vi "Set Protocol Data.vi"(7 "Operation":T1, 8 "error in (no error)":errorcluster, 10 "Protocols.lvlib:Protocol Parent.lvclass":refnum<class "Protocol Parent.lvclass">, 11 "Listener In.lvclass":refnum<class "Listener.lvclass"> caption="Listener") -> (0 "error out":errorcluster, 3 "Listener Out.lvclass":refnum<class "Listener.lvclass">)   [LabVIEW 2019, in "Listener.lvclass"]
uses:
  Listener.lvclass
  Protocol Parent/Protocol Parent.lvclass
  ListenerClassControls/Operation.ctl
  AK TCP/AK TCP.lvclass
  D:/GitRepository/niveristand-instrument-addon-classes/Source/Protocols/TCP/TCP.lvclass
  ListenerClassControls/AK TCP Data Structure.ctl
  ListenerClassControls/Protocol.ctl
  TCP/TCP.lvclass/TCP.ctl
  TCP/TCP.lvclass
  ListenerClassControls/TCP Data Structure.ctl
  UDP/UDP.lvclass
  ListenerClassControls/UDP Data Structure.ctl
  UDP/UDP.lvclass/UDP.ctl
  ListenerClassControls/VISA Data Structure.ctl
  AK RS-xxx/AK RS-xxx.lvclass
  ListenerClassControls/RS-xxx Data Structure.ctl
  ListenerClassControls/RS-xxx To GPIB ConvBox Data Structure.ctl
  TCP/Data Access/Read IP Address.vi
  TCP/Data Access/Read Port.vi
  UDP/Data Access/Read Target IP Address.vi
  UDP/Data Access/Read Local Port.vi
  UDP/Data Access/Read Local IP Address.vi
  UDP/Data Access/Read Target Port.vi
  Constants.vi
  <vilib>/Instr/_visa.llb/VISA Configure Serial Port (Instr).vi
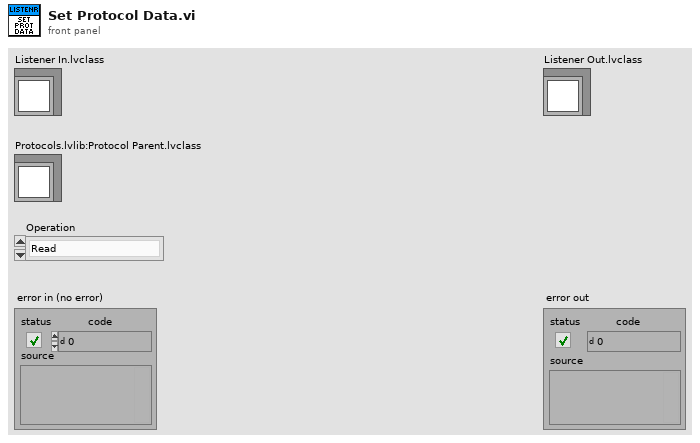
[diagram p1: front panel]
types:
  T1 = typedef "Listener.lvclass/Operation.ctl" = enum16{"Read", "Write"}
  T2 = typedef "Listener.lvclass/Protocol.ctl" = enum16{"RS-XXX", "AK RS-XXX", "VISA", "TCPIP", "AK TCPIP", "UDP", "GPIB ConvBox"}
  T3 = typedef "Listener.lvclass/AK TCP Data Structure.ctl" = cluster{"TCP|IP connection ID":refnum<k5>, "IP Address":string, "Port":u16, "Data":string, "Current Command Code":string}
  T4 = typedef "Listener.lvclass/TCP Data Structure.ctl" = cluster{"TCP|IP connection ID":refnum<k5>, "IP Address":string, "Port":u16, "Data":string}
  T5 = typedef "Listener.lvclass/UDP Data Structure.ctl" = cluster{"UDP connection ID":refnum<k16>, "Local Address":string, "Local Port":u16, "Target IP Address":string, "Target Port":u16, "Data":string}
  T6 = typedef "Listener.lvclass/VISA Data Structure.ctl" = cluster{"Protocol Ref Out":refnum<visa-resource-name>, "Listener Ref Out":refnum<visa-resource-name>, "Data Length":u32, "Data":string}
  T7 = typedef "Listener.lvclass/RS-xxx Data Structure.ctl" = cluster{"Listener Port Ref":refnum<visa-resource-name>, "Protocol Port Ref":refnum<visa-resource-name>, "Virtual COM Port Settings 1":cluster{"Port":string, "Baud Rate":u32, "Data Bits":u16, "Parity":enum16{"None", "Odd", "Even", "Mark", "Space"}, "Stop Bits":u16, "Flow Control":u16, "XON":enum16{"NUL", "SOH", "STX", "ETX", "EOT", "ENQ", "ACK", "BEL", "BS", "HT", "LF", "VT", "FF", "CR", "SO", "SI", "DLE", "DC1", "DC2", "DC3", "DC4", "NAK", "SYN", "ETB", "CAN", "EM", "SUB", "ESC", "FS", "GS", "RS", "US", "SP", "!", "\"", "#", "$", "%", "&", "'", "(", ")", "*", "+", ",", "- (-)", ".", "/", "0", "1", "2", "3", "4", "5", "6", "7", "8", "9", ":", ";", "<", "=", ">", "?", "@", "A", "B", "C", "D", "E", "F", "G", "H", "I", "J", "K", "L", "M", "N", "O", "P", "Q", "R", "S", "T", "U", "V", "W", "X", "Y", "Z", "[", "\\", "]", "^", "_", "`", "a", "b", "c", "d", "e", "f", "g", "h", "i", "j", "k", "l", "m", "n", "o", "p", "q", "r", "s", "t", "u", "v", "w", "x", "y", "z", "{", "|", "}", "~"}, "XOFF":enum16{"NUL", "SOH", "STX", "ETX", "EOT", "ENQ", "ACK", "BEL", "BS", "HT", "LF", "VT", "FF", "CR", "SO", "SI", "DLE", "DC1", "DC2", "DC3", "DC4", "NAK", "SYN", "ETB", "CAN", "EM", "SUB", "ESC", "FS", "GS", "RS", "US", "SP", "!", "\"", "#", "$", "%", "&", "'", "(", ")", "*", "+", ",", "- (-)", ".", "/", "0", "1", "2", "3", "4", "5", "6", "7", "8", "9", ":", ";", "<", "=", ">", "?", "@", "A", "B", "C", "D", "E", "F", "G", "H", "I", "J", "K", "L", "M", "N", "O", "P", "Q", "R", "S", "T", "U", "V", "W", "X", "Y", "Z", "[", "\\", "]", "^", "_", "`", "a", "b", "c", "d", "e", "f", "g", "h", "i", "j", "k", "l", "m", "n", "o", "p", "q", "r", "s", "t", "u", "v", "w", "x", "y", "z", "{", "|", "}", "~"}, "End Read on Termination Character":bool, "End Write on Termination Character":bool, "Termination Character":u8}, "Virtual COM Port Settings 2":cluster{"Port":string, "Baud Rate":u32, "Data Bits":u16, "Parity":enum16{"None", "Odd", "Even", "Mark", "Space"}, "Stop Bits":u16, "Flow Control":u16, "XON":enum16{"NUL", "SOH", "STX", "ETX", "EOT", "ENQ", "ACK", "BEL", "BS", "HT", "LF", "VT", "FF", "CR", "SO", "SI", "DLE", "DC1", "DC2", "DC3", "DC4", "NAK", "SYN", "ETB", "CAN", "EM", "SUB", "ESC", "FS", "GS", "RS", "US", "SP", "!", "\"", "#", "$", "%", "&", "'", "(", ")", "*", "+", ",", "- (-)", ".", "/", "0", "1", "2", "3", "4", "5", "6", "7", "8", "9", ":", ";", "<", "=", ">", "?", "@", "A", "B", "C", "D", "E", "F", "G", "H", "I", "J", "K", "L", "M", "N", "O", "P", "Q", "R", "S", "T", "U", "V", "W", "X", "Y", "Z", "[", "\\", "]", "^", "_", "`", "a", "b", "c", "d", "e", "f", "g", "h", "i", "j", "k", "l", "m", "n", "o", "p", "q", "r", "s", "t", "u", "v", "w", "x", "y", "z", "{", "|", "}", "~"}, "XOFF":enum16{"NUL", "SOH", "STX", "ETX", "EOT", "ENQ", "ACK", "BEL", "BS", "HT", "LF", "VT", "FF", "CR", "SO", "SI", "DLE", "DC1", "DC2", "DC3", "DC4", "NAK", "SYN", "ETB", "CAN", "EM", "SUB", "ESC", "FS", "GS", "RS", "US", "SP", "!", "\"", "#", "$", "%", "&", "'", "(", ")", "*", "+", ",", "- (-)", ".", "/", "0", "1", "2", "3", "4", "5", "6", "7", "8", "9", ":", ";", "<", "=", ">", "?", "@", "A", "B", "C", "D", "E", "F", "G", "H", "I", "J", "K", "L", "M", "N", "O", "P", "Q", "R", "S", "T", "U", "V", "W", "X", "Y", "Z", "[", "\\", "]", "^", "_", "`", "a", "b", "c", "d", "e", "f", "g", "h", "i", "j", "k", "l", "m", "n", "o", "p", "q", "r", "s", "t", "u", "v", "w", "x", "y", "z", "{", "|", "}", "~"}, "End Read on Termination Character":bool, "End Write on Termination Character":bool, "Termination Character":u8}, "Data":string, "Data Length":u32}
  T8 = typedef "Listener.lvclass/RS-xxx To GPIB ConvBox Data Structure.ctl" = cluster{"Protocol Port Ref":refnum<visa-resource-name>, "Listener Port Ref":refnum<visa-resource-name>, "Data":string, "Command Messages Read":string[], "Address":string}
  T9 = typedef "Protocols.lvlib/Protocol Parent.lvclass/Base Protocol Type.ctl" = enum16{"RS-XXX", "VISA", "TCPIP", "UDP", "GPIB ConvBox"}
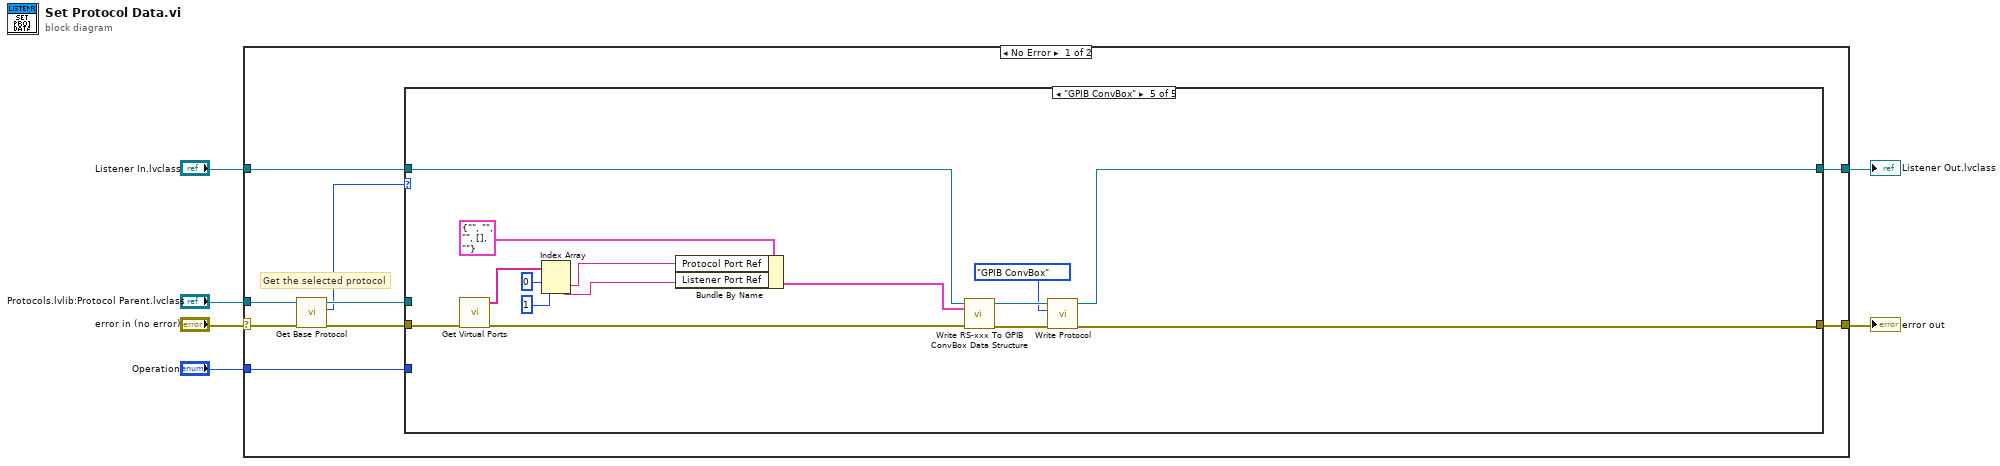
[diagram p0: block diagram]
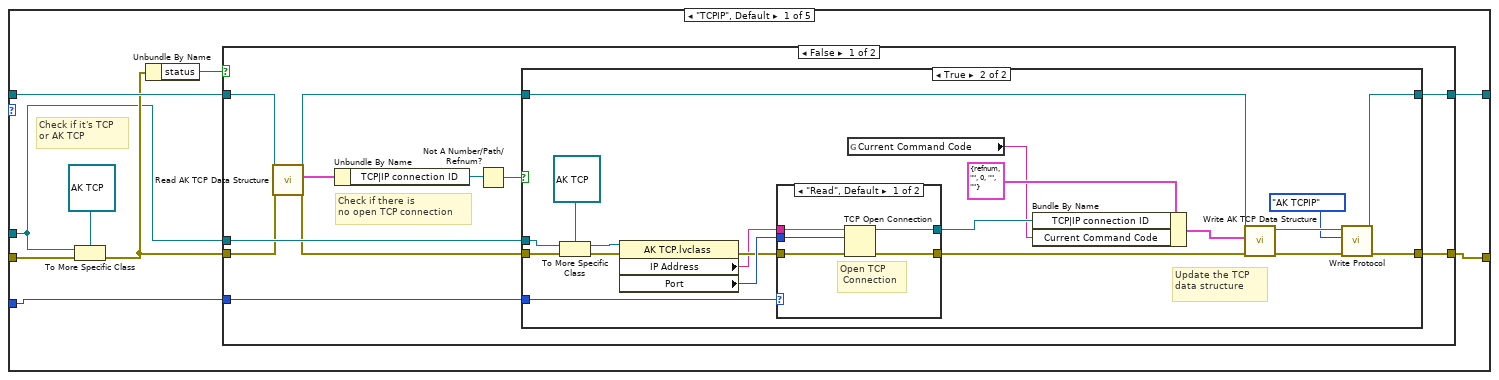
[diagram p2: hidden frame]
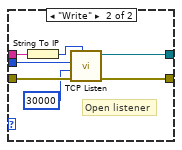
[diagram p4: hidden frame]
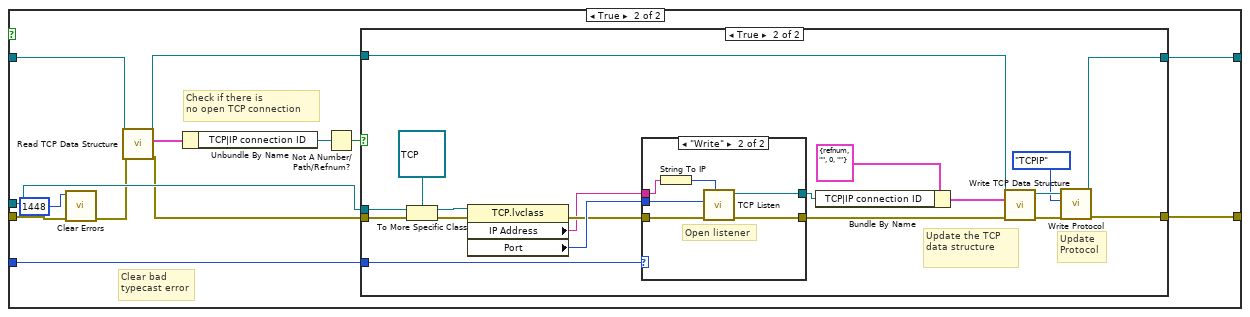
[diagram p5: hidden frame]
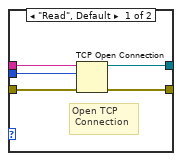
[diagram p7: hidden frame]
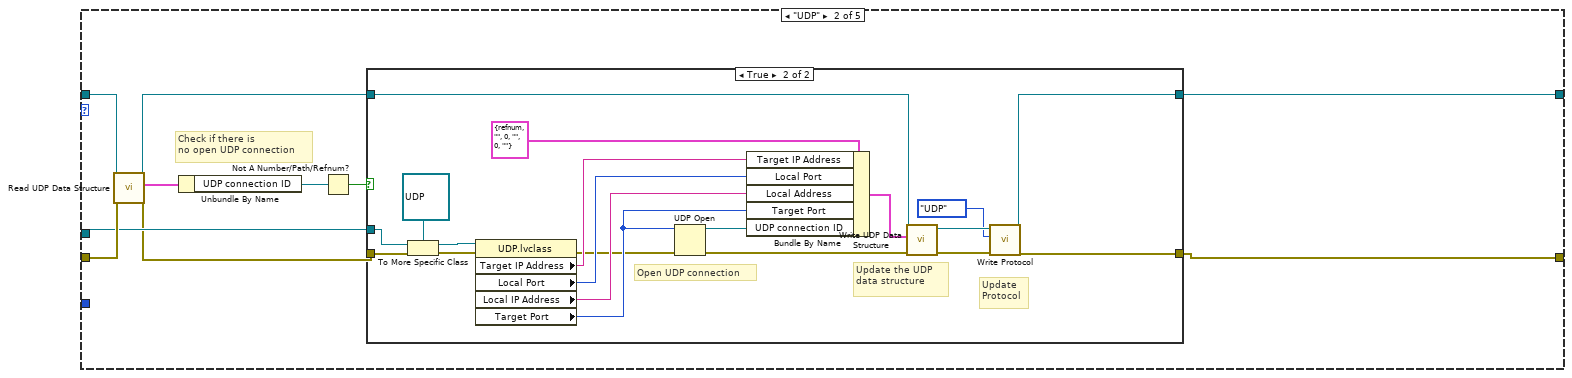
[diagram p8: hidden frame]
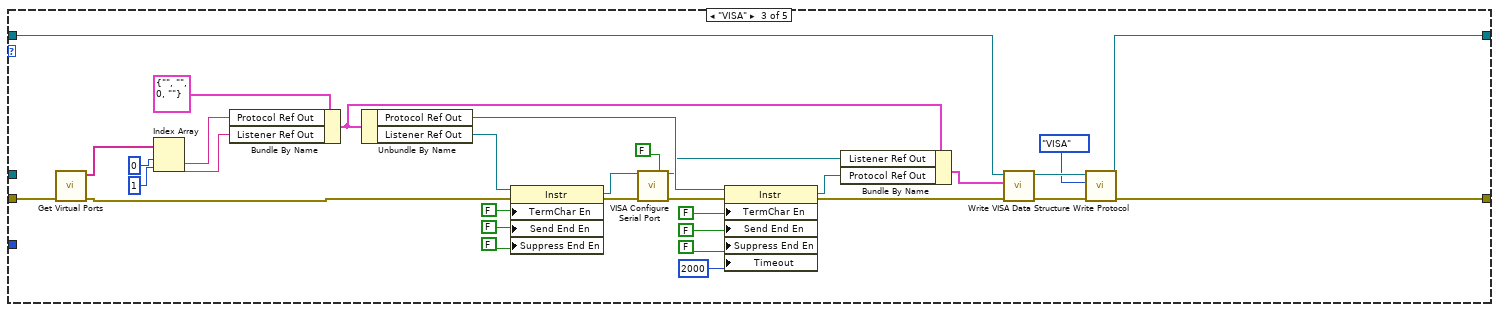
[diagram p10: hidden frame]
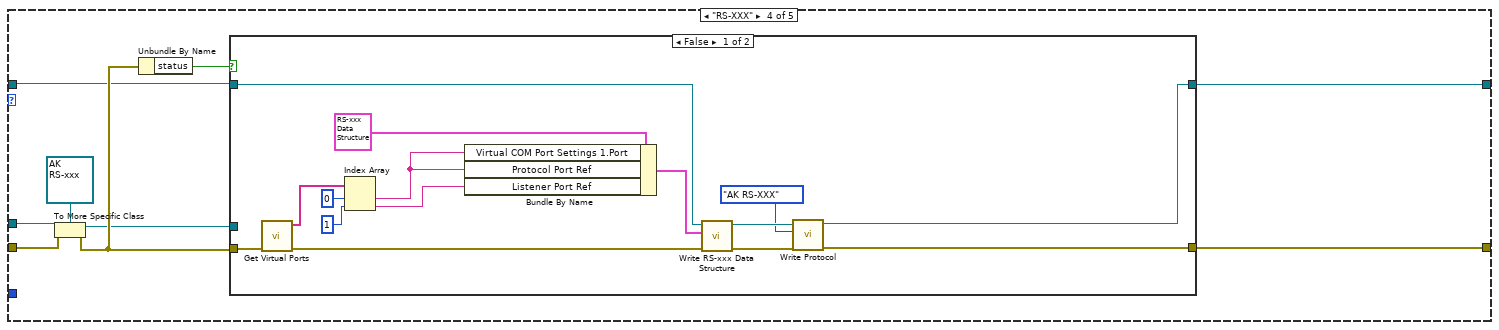
[diagram p11: hidden frame]
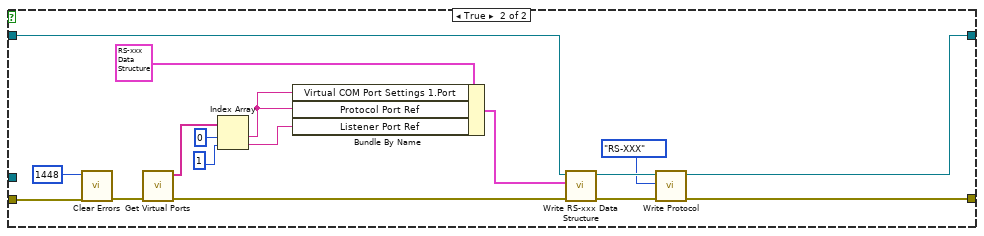
[diagram p12: hidden frame]
diagram:
  n1 = case shown="No Error" "error in (no error)" {
    selector: "error in (no error)" -> [w13 w236]
    tunnel: [w12 w236] -> w5
    tunnel: "Protocols.lvlib:Protocol Parent.lvclass" -> [w14 _]
    tunnel: "Listener In.lvclass" -> [w11 w235]
    tunnel: [w8 w235] -> w2
    tunnel: "Operation" -> [w7 _]
    frame No Error {
      # "Get the selected protocol"
      n2 = call-dynamic "Get Base Protocol.vi"("error in (no error)"=w13, "Protocol Parent in"=w14) -> ("error out"=w10:errorcluster, "Protocol out"=w9:T9, "Protocol Parent out"=w15:refnum<class "Protocol Parent.lvclass">)  [unwired: 7 in]
      n3 = case shown="\"GPIB ConvBox\"" w9 {
        tunnel: w15 -> [w16 w118 _ w180 _]
        tunnel: w10 -> [w20 w120 w178 w187 w234]
        tunnel: [w23 w123 w155 w182 w229] -> w12
        tunnel: w11 -> [w22 w119 w177 w183 w231]
        tunnel: [w24 w124 w174 w181 w227] -> w8
        tunnel: w7 -> [w21 _ _ _ _]
        frame "TCPIP", Default {
          # "Check if it's TCP \nor AK TCP"
          n4 = To More Specific Class(target class=refnum<class "AK TCP.lvclass"> refnum ("Protocols.lvlib:AK TCP.lvclass"), reference=w16, error in=w20) -> (error out=w19:errorcluster)  [unwired: 1 out]
          n5 = Unbundle By Name(w19) -> ("status"=w18:bool)
          n6 = case shown="False" w18 {
            tunnel: w16 -> [w35 w82]
            tunnel: [w34 w81] -> w24
            tunnel: [w33 w80] -> w23
            tunnel: w22 -> [w30 w78]
            tunnel: w19 -> [w28 w77]
            tunnel: w21 -> [w31 w72]
            frame False {
              # "Check if there is \nno open TCP connection"
              n7 = call-dynamic "Read AK TCP Data Structure.vi"("error in (no error)"=w28, "Listener in"=w30) -> ("error out"=w27:errorcluster, "TCP|IP Data Structure"=w26:T3, "Listener out"=w29:refnum<class "Listener.lvclass">)  [unwired: 7 in]
              n8 = Unbundle By Name(w26) -> ("TCP|IP connection ID"=w25:refnum<k5>)
              n9 = Not A Number/Path/Refnum?(number/path/refnum=w25) -> (NaN/Path/Refnum?=w32:bool)
              n10 = case shown="True" w32 {
                tunnel: w35 -> [_ w57]
                tunnel: [w37 w38] -> w34
                tunnel: [w36 w41] -> w33
                tunnel: w27 -> [w36 w54]
                tunnel: w29 -> [w37 w43]
                tunnel: w31 -> [_ w53]
                frame False {
                }
                frame True {
                  # "Update the TCP \ndata structure"
                  n11 = To More Specific Class(target class=refnum<class "AK TCP.lvclass"> refnum ("Protocols.lvlib:AK TCP.lvclass"), reference=w57, error in=w54) -> (specific class reference=w56:refnum<class "AK TCP.lvclass">, error out=w55:errorcluster)
                  n12 = property class="AK TCP.lvclass"(reference=w56, error in=w55) -> (error out=w51:errorcluster, "IP Address"=w50:string, "Port"=w52:u16)  [unwired: 1 out]
                  n13 = case shown="\"Read\", Default" w53 {
                    tunnel: w52 -> [w62 w64]
                    tunnel: w51 -> [w61 w69]
                    tunnel: w50 -> [w60 w68]
                    tunnel: [w59 w65] -> w45
                    tunnel: [w58 w66] -> w49
                    frame "Read", Default {
                      # "Open TCP\n Connection"
                      n14 = TCP Open Connection(address=w60, remote port or service name=w62, error in (no error)=w61) -> (connection ID=w58:refnum<k5>, error out=w59:errorcluster)  [unwired: 2 in]
                    }
                    frame "Write" {
                      # "Open listener"
                      n15 = String To IP(1:w68) -> (0:w67:u32)
                      n16 = call <vilib>:"TCP Listen.vi"("net address"=w67, "error in (no error)"=w69, "timeout ms (wait forever: -1)"=30000, "port"=w64) -> ("error out"=w65:errorcluster, "connection ID"=w66:refnum<k5>)  [unwired: 3 in, 3 out]
                    }
                  }
                  n17 = global read "Constants.vi" "Current Command Code"() -> (w46:string)
                  n18 = Bundle By Name(cluster=T3 {"TCP|IP connection ID"=refnum, "IP Address"="", "Port"=0, "Data"="", "Current Command Code"=""} ("TCP|IP Data Structure"), "TCP|IP connection ID"=w49, "Current Command Code"=w46) -> (w44:T3)
                  n19 = call-dynamic "Write AK TCP Data Structure.vi"("error in (no error)"=w45, "TCP|IP Data Structure"=w44, "Listener in"=w43) -> ("error out"=w42:errorcluster, "Listener out"=w40:refnum<class "Listener.lvclass">)  [unwired: 7 in]
                  n20 = call-dynamic "Write Protocol.vi"("error in (no error)"=w42, "Protocol"=Protocol."AK TCPIP", "Listener in"=w40) -> ("error out"=w41:errorcluster, "Listener out"=w38:refnum<class "Listener.lvclass">)  [unwired: 7 in]
                }
              }
            }
            frame True {
              # "Clear bad \ntypecast error"
              # "Check if there is \nno open TCP connection"
              n21 = call <vilib>:"Clear Errors.vi"("error in (no error)"=w77, "specific error code to clear (0: all)"=1448) -> ("error out"=w71:errorcluster)  [unwired: 4 in, 1 out]
              n22 = call-dynamic "Read TCP Data Structure.vi"("error in (no error)"=w71, "Listener in"=w78) -> ("error out"=w76:errorcluster, "TCP|IP Data Structure"=w75:T4, "Listener out"=w74:refnum<class "Listener.lvclass">)  [unwired: 7 in]
              n23 = Unbundle By Name(w75) -> ("TCP|IP connection ID"=w79:refnum<k5>)
              n24 = Not A Number/Path/Refnum?(number/path/refnum=w79) -> (NaN/Path/Refnum?=w73:bool)
              n25 = case shown="True" w73 {
                tunnel: w82 -> [_ w102]
                tunnel: [w84 w86] -> w81
                tunnel: [w83 w87] -> w80
                tunnel: w76 -> [w83 w98]
                tunnel: w74 -> [w84 w91]
                tunnel: w72 -> [_ w97]
                frame False {
                }
                frame True {
                  # "Update \nProtocol"
                  # "Update the TCP \ndata structure"
                  n26 = To More Specific Class(target class=refnum<class "TCP.lvclass"> refnum ("Protocols.lvlib:TCP.lvclass"), reference=w102, error in=w98) -> (specific class reference=w101:refnum<class "TCP.lvclass">, error out=w100:errorcluster)
                  n27 = property class="TCP.lvclass"(reference=w101, error in=w100) -> (error out=w95:errorcluster, "IP Address"=w94:string, "Port"=w96:u16)  [unwired: 1 out]
                  n28 = case shown="\"Write\"" w97 {
                    tunnel: w96 -> [w108 w113]
                    tunnel: w95 -> [w107 w114]
                    tunnel: w94 -> [w106 w112]
                    tunnel: [w105 w109] -> w92
                    tunnel: [w104 w110] -> w93
                    frame "Read", Default {
                      # "Open TCP\n Connection"
                      n29 = TCP Open Connection(address=w106, remote port or service name=w108, error in (no error)=w107) -> (connection ID=w104:refnum<k5>, error out=w105:errorcluster)  [unwired: 2 in]
                    }
                    frame "Write" {
                      # "Open listener"
                      n30 = String To IP(1:w112) -> (0:w111:u32)
                      n31 = call <vilib>:"TCP Listen.vi"("net address"=w111, "error in (no error)"=w114, "port"=w113) -> ("error out"=w109:errorcluster, "connection ID"=w110:refnum<k5>)  [unwired: 4 in, 3 out]
                    }
                  }
                  n32 = Bundle By Name(cluster=T4 {"TCP|IP connection ID"=refnum, "IP Address"="", "Port"=0, "Data"=""} ("TCP|IP Data Structure"), "TCP|IP connection ID"=w93) -> (w90:T4)
                  n33 = call-dynamic "Write TCP Data Structure.vi"("error in (no error)"=w92, "TCP|IP Data Structure"=w90, "Listener in"=w91) -> ("error out"=w89:errorcluster, "Listener out"=w88:refnum<class "Listener.lvclass">)  [unwired: 7 in]
                  n34 = call-dynamic "Write Protocol.vi"("error in (no error)"=w89, "Protocol"=Protocol."TCPIP", "Listener in"=w88) -> ("error out"=w87:errorcluster, "Listener out"=w86:refnum<class "Listener.lvclass">)  [unwired: 7 in]
                }
              }
            }
          }
        }
        frame "UDP" {
          # "Check if there is \nno open UDP connection"
          n35 = call-dynamic "Read UDP Data Structure.vi"("error in (no error)"=w120, "Listener in"=w119) -> ("error out"=w116:errorcluster, "UDP Data Structure"=w117:T5, "Listener out"=w115:refnum<class "Listener.lvclass">)  [unwired: 7 in]
          n36 = Unbundle By Name(w117) -> ("UDP connection ID"=w121:refnum<k16>)
          n37 = Not A Number/Path/Refnum?(number/path/refnum=w121) -> (NaN/Path/Refnum?=w122:bool)
          n38 = case shown="True" w122 {
            tunnel: w116 -> [w126 w146]
            tunnel: w118 -> [_ w144]
            tunnel: w115 -> [w125 w133]
            tunnel: [w125 w127] -> w124
            tunnel: [w126 w128] -> w123
            frame False {
            }
            frame True {
              # "Update \nProtocol"
              # "Update the UDP \ndata structure"
              # "Open UDP connection"
              n39 = To More Specific Class(target class=refnum<class "UDP.lvclass"> refnum ("Protocols.lvlib:UDP.lvclass"), reference=w144, error in=w146) -> (specific class reference=w138:refnum<class "UDP.lvclass">, error out=w143:errorcluster)
              n40 = property class="UDP.lvclass"(reference=w138, error in=w143) -> (error out=w136:errorcluster, "Target IP Address"=w142:string, "Local Port"=w141:u16, "Local IP Address"=w140:string, "Target Port"=w137:u16)  [unwired: 1 out]
              n41 = UDP Open(8:w136, 11:w137) -> (port=w135:refnum<k16>, 0:w134:errorcluster)  [unwired: 3 in, 1 out]
              n42 = Bundle By Name(cluster=T5 {"UDP connection ID"=refnum, "Local Address"="", "Local Port"=0, "Target IP Address"="", "Target Port"=0, "Data"=""} ("UDP Data Structure"), "Target IP Address"=w142, "Local Port"=w141, "Local Address"=w140, "Target Port"=w137, "UDP connection ID"=w135) -> (w132:T5)
              n43 = call-dynamic "Write UDP Data Structure.vi"("error in (no error)"=w134, "UDP Data Structure"=w132, "Listener in"=w133) -> ("error out"=w131:errorcluster, "Listener out"=w130:refnum<class "Listener.lvclass">)  [unwired: 7 in]
              n44 = call-dynamic "Write Protocol.vi"("error in (no error)"=w131, "Protocol"=Protocol."UDP", "Listener in"=w130) -> ("error out"=w128:errorcluster, "Listener out"=w127:refnum<class "Listener.lvclass">)  [unwired: 7 in]
            }
          }
        }
        frame "VISA" {
          n45 = call "Get Virtual Ports.vi"("error in (no error)"=w178) -> ("error out"=w154:errorcluster, "Serial Ports out"=w170:string[])  [unwired: 9 in]
          n46 = Index Array(array=w170, index #1=0 ("index"), index #2=1 ("index")) -> (element #1=w169:string, element #2=w168:string)
          n47 = Bundle By Name(cluster=T6 {"Protocol Ref Out"="", "Listener Ref Out"="", "Data Length"=0, "Data"=""}, "Protocol Ref Out"=w169, "Listener Ref Out"=w168) -> (w165:T6)
          n48 = Unbundle By Name(w165) -> ("Protocol Ref Out"=w153:refnum<visa-resource-name>, "Listener Ref Out"=w166:refnum<visa-resource-name>)
          n49 = property class="Instr"(reference=w166, error in=w154, "TermChar En"=FALSE ("Message Based Settings:Termination Character Enable"), "Send End En"=FALSE ("Message Based Settings:Send End Enable"), "Suppress End En"=FALSE ("Message Based Settings:Suppress End Enable")) -> (reference out=w150:refnum<visa-resource-name>, error out=w152:errorcluster)
          n50 = call-poly "VISA Configure Serial Port"("VISA resource name"=w150, "Enable Termination\nChar (T)"=FALSE ("Enable Termination\nChar (T)"), "error in (no error)"=w152) -> ("VISA resource name out"=w148:refnum<visa-resource-name>, "error out"=w151:errorcluster)  [unwired: 11 in]
          n51 = property class="Instr"(reference=w153, error in=w151, "TermChar En"=FALSE ("Message Based Settings:Termination Character Enable"), "Send End En"=FALSE ("Message Based Settings:Send End Enable"), "Suppress End En"=FALSE ("Message Based Settings:Suppress End Enable"), "Timeout"=u32 2000 ("General Settings:Timeout Value")) -> (reference out=w149:refnum<visa-resource-name>, error out=w147:errorcluster)
          n52 = Bundle By Name(cluster=w165, "Listener Ref Out"=w148, "Protocol Ref Out"=w149) -> (w164:T6)
          n53 = call-dynamic "Write VISA Data Structure.vi"("error in (no error)"=w147, "VISA Data Structure"=w164, "Listener in"=w177) -> ("error out"=w176:errorcluster, "Listener out"=w175:refnum<class "Listener.lvclass">)  [unwired: 7 in]
          n54 = call-dynamic "Write Protocol.vi"("error in (no error)"=w176, "Protocol"=Protocol."VISA", "Listener in"=w175) -> ("error out"=w155:errorcluster, "Listener out"=w174:refnum<class "Listener.lvclass">)  [unwired: 7 in]
        }
        frame "RS-XXX" {
          n55 = To More Specific Class(target class=refnum<class "AK RS-xxx.lvclass"> refnum ("Protocols.lvlib:AK RS-xxx.lvclass"), reference=w180, error in=w187) -> (specific class reference=w179:refnum<class "AK RS-xxx.lvclass">, error out=w184:errorcluster)
          n56 = Unbundle By Name(w184) -> ("status"=w185:bool)
          n57 = case shown="False" w185 {
            tunnel: w184 -> [w202 w219]
            tunnel: w183 -> [w201 w215]
            tunnel: [w199 w213] -> w182
            tunnel: [w197 w214] -> w181
            tunnel: w179 -> [_ _]
            frame False {
              n58 = call "Get Virtual Ports.vi"("error in (no error)"=w202) -> ("error out"=w191:errorcluster, "Serial Ports out"=w192:string[])  [unwired: 9 in]
              n59 = Index Array(array=w192, index #1=0 ("index"), index #2=1 ("index")) -> (element #1=w188:string, element #2=w190:string)
              n60 = Bundle By Name(cluster=T7 {"Listener Port Ref"="", "Protocol Port Ref"="", "Virtual COM Port Settings 1"={"Port"="COM1", "Baud Rate"=9600, "Data Bits"=8, "Parity"=enum."None", "Stop Bits"=10, "Flow Control"=0, "XON"=enum."DC1", "XOFF"=enum."DC3", "End Read on Termination Character"=FALSE, "End Write on Termination Character"=FALSE, "Termination Character"=10}, "Virtual COM Port Settings 2"={"Port"="COM1", "Baud Rate"=9600, "Data Bits"=8, "Parity"=enum."None", "Stop Bits"=10, "Flow Control"=0, "XON"=enum."DC1", "XOFF"=enum."DC3", "End Read on Termination Character"=FALSE, "End Write on Termination Character"=FALSE, "Termination Character"=10}, "Data"="", "Data Length"=0} ("RS-xxx Data Structure"), "Virtual COM Port Settings 1.Port"=w188, "Protocol Port Ref"=w188, "Listener Port Ref"=w190) -> (w189:T7)
              n61 = call-dynamic "Write RS-xxx Data Structure.vi"("error in (no error)"=w191, "RS-xxx Data Structure"=w189, "Listener in"=w201) -> ("error out"=w200:errorcluster, "Listener out"=w198:refnum<class "Listener.lvclass">)  [unwired: 7 in]
              n62 = call-dynamic "Write Protocol.vi"("error in (no error)"=w200, "Protocol"=Protocol."AK RS-XXX", "Listener in"=w198) -> ("error out"=w199:errorcluster, "Listener out"=w197:refnum<class "Listener.lvclass">)  [unwired: 7 in]
            }
            frame True {
              n63 = call <vilib>:"Clear Errors.vi"("error in (no error)"=w219, "specific error code to clear (0: all)"=1448) -> ("error out"=w211:errorcluster)  [unwired: 4 in, 1 out]
              n64 = call "Get Virtual Ports.vi"("error in (no error)"=w211) -> ("error out"=w204:errorcluster, "Serial Ports out"=w208:string[])  [unwired: 9 in]
              n65 = Index Array(array=w208, index #1=0 ("index"), index #2=1 ("index")) -> (element #1=w206:string, element #2=w207:string)
              n66 = Bundle By Name(cluster=T7 {"Listener Port Ref"="", "Protocol Port Ref"="", "Virtual COM Port Settings 1"={"Port"="COM1", "Baud Rate"=9600, "Data Bits"=8, "Parity"=enum."None", "Stop Bits"=10, "Flow Control"=0, "XON"=enum."DC1", "XOFF"=enum."DC3", "End Read on Termination Character"=FALSE, "End Write on Termination Character"=FALSE, "Termination Character"=10}, "Virtual COM Port Settings 2"={"Port"="COM1", "Baud Rate"=9600, "Data Bits"=8, "Parity"=enum."None", "Stop Bits"=10, "Flow Control"=0, "XON"=enum."DC1", "XOFF"=enum."DC3", "End Read on Termination Character"=FALSE, "End Write on Termination Character"=FALSE, "Termination Character"=10}, "Data"="", "Data Length"=0} ("RS-xxx Data Structure"), "Virtual COM Port Settings 1.Port"=w206, "Protocol Port Ref"=w206, "Listener Port Ref"=w207) -> (w203:T7)
              n67 = call-dynamic "Write RS-xxx Data Structure.vi"("error in (no error)"=w204, "RS-xxx Data Structure"=w203, "Listener in"=w215) -> ("error out"=w218:errorcluster, "Listener out"=w217:refnum<class "Listener.lvclass">)  [unwired: 7 in]
              n68 = call-dynamic "Write Protocol.vi"("error in (no error)"=w218, "Protocol"=Protocol."RS-XXX", "Listener in"=w217) -> ("error out"=w213:errorcluster, "Listener out"=w214:refnum<class "Listener.lvclass">)  [unwired: 7 in]
            }
          }
        }
        frame "GPIB ConvBox" {
          n69 = call "Get Virtual Ports.vi"("error in (no error)"=w234) -> ("error out"=w223:errorcluster, "Serial Ports out"=w222:string[])  [unwired: 9 in]
          n70 = Index Array(array=w222, index #1=0 ("index"), index #2=1 ("index")) -> (element #1=w221:string, element #2=w220:string)
          n71 = Bundle By Name(cluster=T8 {"Protocol Port Ref"="", "Listener Port Ref"="", "Data"="", "Command Messages Read"=[], "Address"=""}, "Protocol Port Ref"=w221, "Listener Port Ref"=w220) -> (w232:T8)
          n72 = call-dynamic "Write RS-xxx To GPIB ConvBox Data Structure.vi"("error in (no error)"=w223, "RS-xxx To GPIB ConvBox Data Structure"=w232, "Listener in"=w231) -> ("error out"=w230:errorcluster, "Listener out"=w228:refnum<class "Listener.lvclass">)  [unwired: 7 in]
          n73 = call-dynamic "Write Protocol.vi"("error in (no error)"=w230, "Protocol"=Protocol."GPIB ConvBox", "Listener in"=w228) -> ("error out"=w229:errorcluster, "Listener out"=w227:refnum<class "Listener.lvclass">)  [unwired: 7 in]
        }
      }
    }
    frame Error {
    }
  }
  "Listener Out.lvclass" <- w2
  "error out" <- w5
